vi "simulateImageAcqusition.vi"() -> (3 "objRef":dbl[][](array[numeric]), 5 "imgRaw":dbl[][](array[numeric]))   [LabVIEW 2012]
uses:
  <vilib>/Utility/error.llb/DialogType.ctl
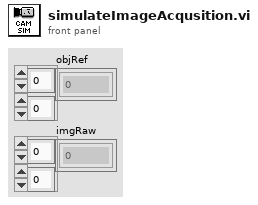
[diagram p1: front panel]
types:
  T1 = typedef "DialogType.ctl" = u16
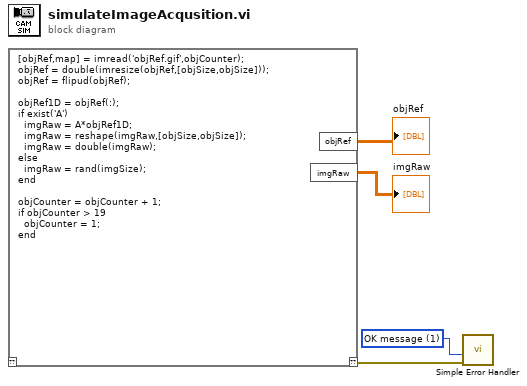
[diagram p0: block diagram]
diagram:
  w2 = T1 1 items=["no dialog", "OK message", "continue or stop message", "OK message + warnings", "continue/stop + warnings"] ("type of dialog (OK msg:1)")
  n1 = script code="[objRef,map] = imread('objRef.gif',objCounter);\nobjRef = double(imresize(objRef,[objSize,objSize]));\nobjRef = flipud(objRef);\n\nobjRef1D = objRef(:);\nif exist('A')\n  imgRaw = A*objRef1D;\n  imgRaw = reshape(imgRaw,[objSize,objSize]);\n  imgRaw = double(imgRaw);\nelse\n  imgRaw = rand(imgSize); \nend\n\nobjCounter = objCounter + 1;\nif objCounter > 19\n  objCounter = 1;\nend"() -> ("??"=w3:errorcluster, "objRef"=→"objRef":dbl[][], "imgRaw"=→"imgRaw":dbl[][])  [unwired: 1 in]
  n2 = call <vilib>:"Simple Error Handler.vi"("type of dialog (OK msg:1)"=w2, "error in (no error)"=w3) -> ()  [unwired: 3 in, 5 out]
